vi "BGA244_get_gas_type.vi"(8 "error in":errorcluster, 11 "VISA in":refnum<visa-resource-name>) -> (0 "error out":errorcluster, 1 "gas 2":string, 2 "gas 1":string, 3 "VISA out":refnum<visa-resource-name>, 4 "status":bool)   [LabVIEW 2019]
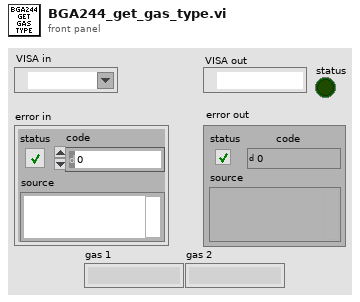
[diagram p1: front panel]
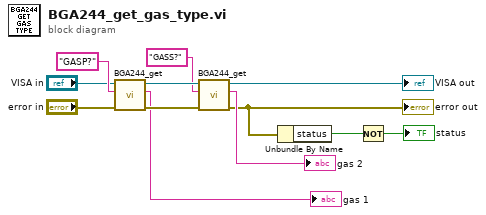
[diagram p0: block diagram]
diagram:
  n1 = call "BGA244_get.vi"("error in"="error in", "string in"="GASP?" ("string"), "VISA in"="VISA in") -> ("error out"=w7:errorcluster, "string out"=→"gas 1":string, "VISA out"=w9:refnum<visa-resource-name>)  [unwired: 6 in]
  n2 = call "BGA244_get.vi"("error in"=w7, "string in"="GASS?" ("string"), "VISA in"=w9) -> ("error out"=w3:errorcluster, "string out"=→"gas 2":string, "VISA out"=→"VISA out":refnum<visa-resource-name>)  [unwired: 6 in]
  "error out" <- w3
  n3 = Unbundle By Name(w3) -> ("status"=w2:bool)
  n4 = Not(x=w2) -> (.not. x?=→"status":bool)
